vi "Set Power Failure Delay.vi"(1 "Delay before Power Failure Closure":u16, 2 "Boolean":bool) -> (0 "result string":string)   [LabVIEW 2009]
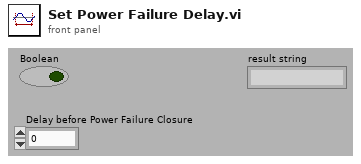
[diagram p1: front panel]
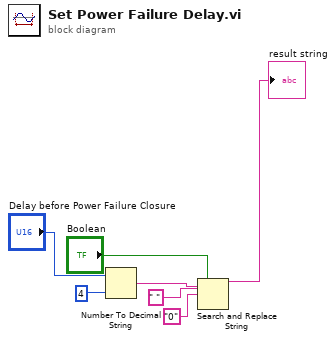
[diagram p0: block diagram]
diagram:
  n1 = Number To Decimal String(number="Delay before Power Failure Closure", width (-)=i16 4) -> (decimal integer string=w6:string)
  n2 = Search and Replace String(replace all?="Boolean", input string=w6, search string=" ", replace string="0") -> (result string=→"result string":string)  [unwired: 4 in, 3 out]
